vi "svfa_Scaled Time Domain Window (N Ch).vi"(0 "Scaled signal(s)":waveform(dbl)[](array[waveform]), 5 "window":T1=1 items=["None"=0, "Hanning"=1, "Hamming"=2, "Blackman-Harris"=3, "Exact Blackman"=4, "Blackman"=5, "Flat Top"=6, "4 Term B-Harris "=7, "7 Term B-Harris"=8, "Low Sidelobe"=9, "Force"=64, "Exponential"=65, "Blackman Nuttall"=11, "Triangle"=30, "Bartlett-Hanning"=31, "Bohman"=32, "Parzen"=33, "Welch"=34, "Kaiser"=60, "Dolph-Chebyshev"=61, "Gaussian"=62], 7 "window parameter":dbl=nan format="%0.2f", 11 "error in (no error)":errorcluster) -> (4 "Windowed Waveform(s)":waveform(dbl)[](array[waveform]), 6 "window":T1 items=["None"=0, "Hanning"=1, "Hamming"=2, "Blackman-Harris"=3, "Exact Blackman"=4, "Blackman"=5, "Flat Top"=6, "4 Term B-Harris "=7, "7 Term B-Harris"=8, "Low Sidelobe"=9, "Force"=64, "Exponential"=65, "Blackman Nuttall"=11, "Triangle"=30, "Bartlett-Hanning"=31, "Bohman"=32, "Parzen"=33, "Welch"=34, "Kaiser"=60, "Dolph-Chebyshev"=61, "Gaussian"=62], 8 "window length":i32, 13 "window constants":cluster{"ENBW":dbl, "CG":dbl} {"CG" format="%.2f"; "ENBW" format="%.2f"}, 15 "error out":errorcluster)   [LabVIEW 2017]
doc: "Applies the selected window to the time-domain signal. The VI scales the result so that when the power or amplitude spectrum of the windowed waveform is computed, all windows provide the same level within the accuracy constraints of the window."
uses:
  <vilib>/addons/_NISVFA/_Shared subVIs/Controls/svc_Window.ctl
  <vilib>/addons/_NISVFA/_Shared subVIs/Windowing/svfa_Scaled Time Domain Window (Array).vi
  <vilib>/Analysis/4window.llb/Force Window.vi
  <vilib>/Analysis/4window.llb/Force Window (DBL).vi
  <vilib>/Analysis/4window.llb/Exponential Window.vi
  <vilib>/Analysis/4window.llb/Exponential Window (DBL).vi
  <vilib>/Utility/error.llb/Error Cluster From Error Code.vi
  <vilib>/Analysis/0measdsp.llb/Scaled Time Domain Window.vi
  <vilib>/Analysis/0measdsp.llb/Scaled Time Domain Window (DBL).vi
  <vilib>/addons/_NISVFA/_Spectrum Processing/subVIs/svfa_Spectrum Info Window to windowTd Type Def.vi
  <vilib>/addons/_NISVFA/_Shared subVIs/Common/svc_Window Parameters.vi
  <vilib>/addons/_NISVFA/_Shared subVIs/Common/svc_Get Window Info.vi
panel:
  # "Scaled Time Domain Window"
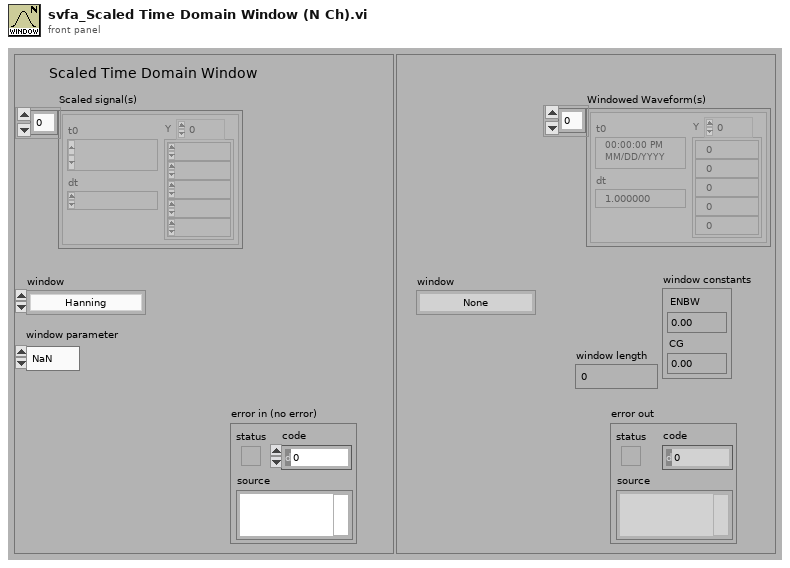
[diagram p1: front panel]
types:
  T1 = typedef "svc_Window.ctl" = u32
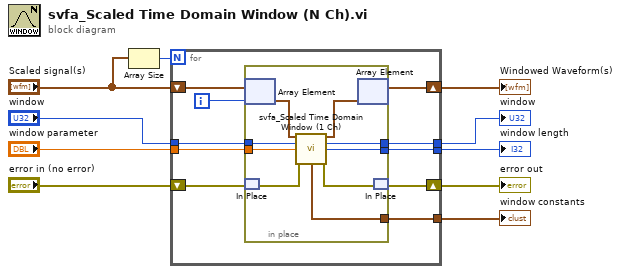
[diagram p0: block diagram]
diagram:
  n1 = Array Size(array="Scaled signal(s)") -> (size(s)=w1:i32)
  n2 = for {
    N: w1 -> [_]
    shift-right: [w13] -> w7
    shift-left: "Scaled signal(s)" -> [w15]
    tunnel: "window" -> [w20]
    tunnel: [w19] -> w3
    tunnel: [w18] -> w4
    shift-right: [w11] -> w5
    shift-left: "error in (no error)" -> [w12]
    tunnel: [w17] -> w6
    tunnel: "window parameter" -> [w16]
    i -> [w14]
    n3 = in-place {
      in-place-border: w20 -> [w29]
      in-place-border: [w28] -> w19
      in-place-border: [w27] -> w18
      in-place-border: [w26] -> w17
      in-place-border: w16 -> [w25]
      n4 = in-place-array #1(w15, w14) -> (w24:waveform(dbl))
      n5 = in-place-match #2(w12) -> (w22:errorcluster)
      n6 = call <vilib>:"svfa_Scaled Time Domain Window (1 Ch).vi"("Signal in [X]"=w24, "window"=w29, "window parameter"=w25, "error in"=w22) -> ("Windowed Waveform"=w23:waveform(dbl), "dup window"=w26:T1, "window length"=w27:i32, "window constants"=w28:cluster{"ENBW":dbl, "CG":dbl}, "error out"=w21:errorcluster)  [unwired: 6 in, 1 out]
      n7 = in-place-array #1(w23) -> (w13:waveform(dbl)[])  [unwired: 1 out]
      n8 = in-place-match #2(w21) -> (w11:errorcluster)
    }
  }
  "error out" <- w5
  "window constants" <- w3
  "Windowed Waveform(s)" <- w7
  "window" <- w6
  "window length" <- w4
